vi "GetMethods.vi"(0 "ClassReader in":refnum<class "ClassReader.lvclass">, 5 "error in (no error)":errorcluster) -> (14 "ClassReader out":refnum<class "ClassReader.lvclass">, 15 "Methods":T1[](array[typedef]), 16 "Constructor/CreateIndex":i32, 19 "error out":errorcluster)   [LabVIEW 2014, in "ClassReader.lvclass"]
uses:
  <resource>/Framework/Providers/Open_GDS/ClassProviders/Provider_BaseClassInterface/ClassReader_class/ClassReader.lvclass
  <resource>/Framework/Providers/Open_GDS/ClassProviders/Provider_BaseClassInterface/Types/ClassTypes_MethodType.ctl
  <resource>/Framework/Providers/Open_GDS/ClassProviders/Provider_BaseClassInterface/ClassReader_class/ClassReader.lvclass/ClassReader.ctl
  <resource>/Framework/Providers/Open_GDS/UML/UMLEditor/UMLEditor_VisibilityType.ctl
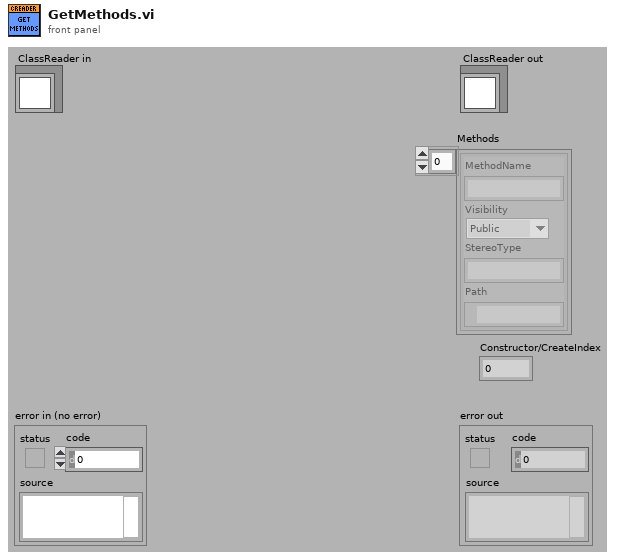
[diagram p1: front panel]
types:
  T1 = typedef "ClassTypes_MethodType.ctl" = cluster{"MethodName":string, "Visibility":enum16{"Public", "Private", "Protected"}, "StereoType":string, "Path":path}
  T2 = typedef "UMLEditor_VisibilityType.ctl" = enum16{"Public", "Private", "Protected"}
  T3 = typedef "Librarian File Info Out.ctl" = cluster{"creation date":u32, "last mod date":u32, "type":string, "creator":string, "LV version":i32, "size":i32, "top level":bool}
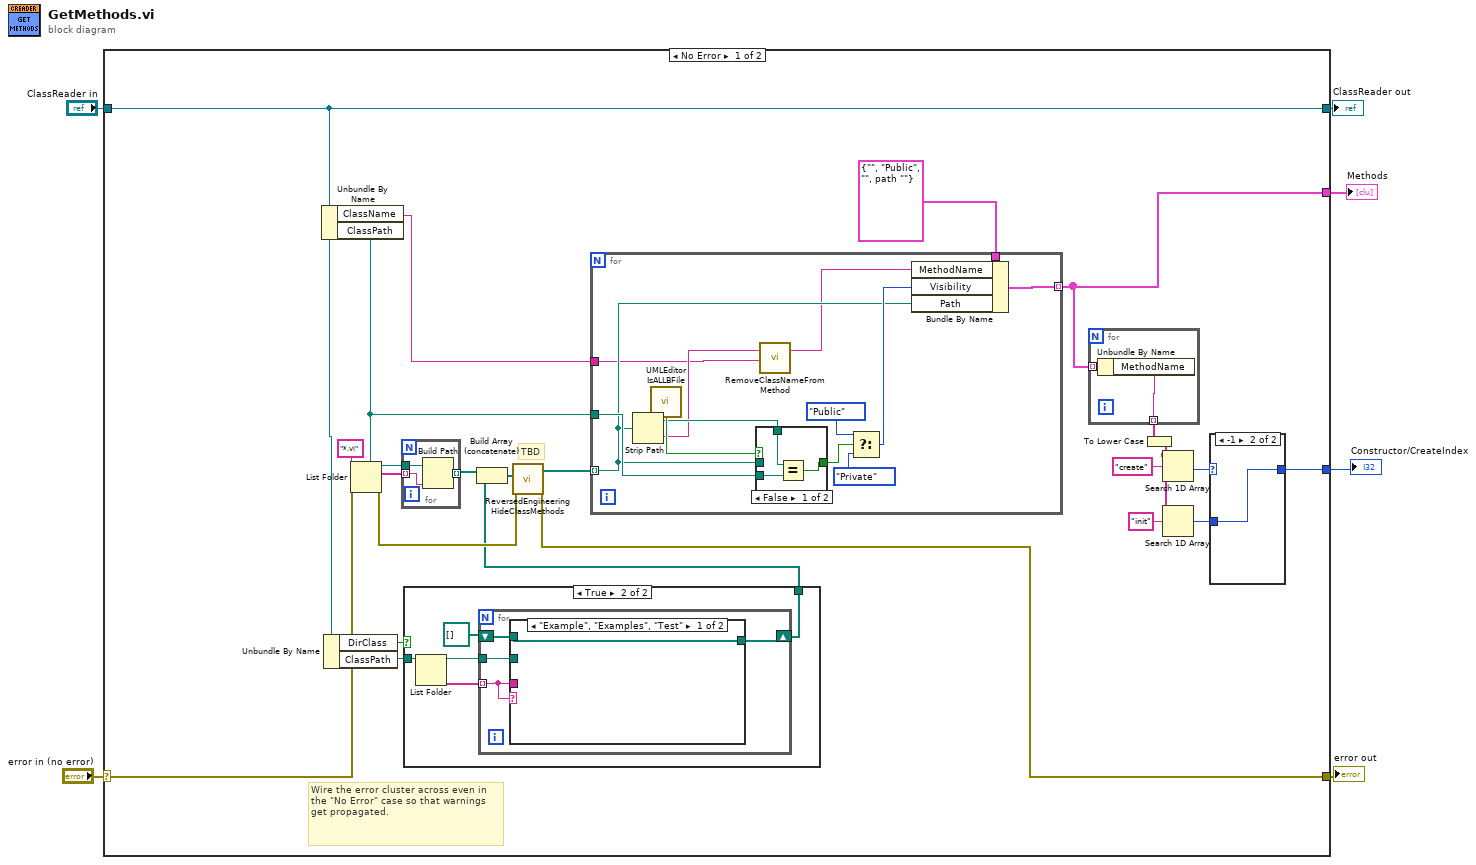
[diagram p0: block diagram]
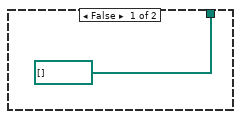
[diagram p3: hidden frame]
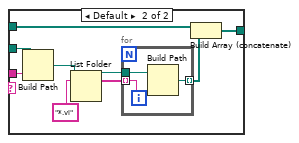
[diagram p4: hidden frame]
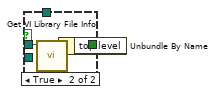
[diagram p5: hidden frame]
diagram:
  n1 = case shown="No Error" "error in (no error)" {
    selector: "error in (no error)" -> [w18 w81]
    tunnel: [w15 w81] -> w5
    tunnel: [w17 w80] -> w3
    tunnel: "ClassReader in" -> [w17 w80]
    tunnel: [w8 _] -> w2
    tunnel: [w7 _] -> w1
    frame No Error {
      # "TBD"
      # "Wire the error cluster across even in the \"No Error\" case so that warnings get propagated."
      n2 = Unbundle By Name(w17) -> ("ClassName"=w22:string, "ClassPath"=w19:path)
      n3 = Unbundle By Name(w17) -> ("DirClass"=w24:bool, "ClassPath"=w23:path)
      n4 = List Folder(path=w19, pattern="*.vi", error in=w18) -> (path out=w30:path, filenames=w29:string[], error out=w26:errorcluster)  [unwired: 1 in, 1 out]
      n5 = for {
        tunnel: w30 -> [w79]
        tunnel: w29 -> [w77] mode=indexing
        tunnel: [w78] -> w28 mode=indexing
        n6 = Build Path(base path=w79, name or relative path=w77) -> (appended path=w78:path)
      }
      n7 = case shown="True" w24 {
        tunnel: w23 -> [_ w40]
        tunnel: [path[] [] w37] -> w21
        frame False {
        }
        frame True {
          n8 = List Folder(path=w40) -> (path out=w39:path, folder names=w38:string[])  [unwired: 3 in, 2 out]
          n9 = for {
            tunnel: w39 -> [w44]
            tunnel: w38 -> [w41] mode=indexing
            shift-right: [w42] -> w37
            shift-left: path[] [] -> [w43]
            n10 = case shown="\"Example\", \"Examples\", \"Test\"" w41 {
              tunnel: w44 -> [_ w51]
              tunnel: w41 -> [_ w50]
              tunnel: w43 -> [w45 w48]
              tunnel: [w45 w47] -> w42
              frame "Example", "Examples", "Test" {
              }
              frame Default {
                n11 = Build Path(base path=w51, name or relative path=w50) -> (appended path=w49:path)
                n12 = List Folder(path=w49, pattern="*.vi") -> (path out=w53:path, filenames=w54:string[])  [unwired: 2 in, 2 out]
                n13 = for {
                  tunnel: w53 -> [w57]
                  tunnel: w54 -> [w55] mode=indexing
                  tunnel: [w56] -> w46 mode=indexing
                  n14 = Build Path(base path=w57, name or relative path=w55) -> (appended path=w56:path)
                }
                n15 = Build Array (concatenate)(w48, w46) -> (w47:path[])
              }
            }
          }
        }
      }
      n16 = Build Array (concatenate)(w28, w21) -> (w20:path[])
      n17 = call <resource>:"ReversedEngineering HideClassMethods.vi"("Item Paths"=w20, "error in (no error)"=w26) -> ("Item Paths filtered"=w27:path[], "error out"=w15:errorcluster)  [unwired: 16 in]
      n18 = for {
        tunnel: w27 -> [w62] mode=indexing
        tunnel: w22 -> [w58]
        tunnel: w19 -> [w68]
        tunnel: T1 {"MethodName"="", "Visibility"=enum."Public", "StereoType"="", "Path"=path ""} ("Method") -> [w64]
        tunnel: [w61] -> w8 mode=indexing
        n19 = Strip Path(path=w62) -> (stripped path=w69:path, name=w60:string)
        n20 = call <resource>:"UMLEditor IsALLBFile.vi"("path"=w69) -> ("path to VI library?"=w70:bool)
        n21 = case shown="False" w70 {
          tunnel: [w71 w75] -> w67
          tunnel: w62 -> [_ w74]
          tunnel: w69 -> [w73 _]
          tunnel: w68 -> [w72 _]
          frame False {
            n22 = Equal?(x=w73, y=w72) -> (x = y?=w71:bool)
          }
          frame True {
            n23 = call <vilib>:"Get VI Library File Info.vi"("path"=w74) -> ("file information"=w76:T3)  [unwired: 9 in, 1 out]
            n24 = Unbundle By Name(w76) -> ("top level"=w75:bool)
          }
        }
        n25 = call <resource>:"RemoveClassNameFromMethod.vi"("MethodVINameIn"=w60, "ClassName"=w58) -> ("MethodVINameOut"=w59:string)  [unwired: 17 in]
        n26 = Select(t=UMLEditor_VisibilityType."Public" ("Enum"), s=w67, f=UMLEditor_VisibilityType."Private" ("Enum")) -> (s? t:f=w63:T2)
        n27 = Bundle By Name(cluster=w64, "MethodName"=w59, "Visibility"=w63, "Path"=w62) -> (w61:T1)
      }
      n28 = for {
        tunnel: w8 -> [w34] mode=indexing
        tunnel: [w33] -> w14 mode=indexing
        n29 = Unbundle By Name(w34) -> ("MethodName"=w33:string)
      }
      n30 = To Lower Case(string=w14) -> (all lower case string=w12:string[])
      n31 = Search 1D Array(1D array=w12, element="create") -> (index of element=w10:i32)  [unwired: 1 in]
      n32 = Search 1D Array(1D array=w12, element="init") -> (index of element=w9:i32)  [unwired: 1 in]
      n33 = case shown="-1" w10 {
        selector: w10 -> [w31 _]
        tunnel: [w31 w32] -> w7
        tunnel: w9 -> [_ w32]
        frame Default {
        }
        frame -1 {
        }
      }
    }
    frame Error {
    }
  }
  "error out" <- w5
  "ClassReader out" <- w3
  "Methods" <- w2
  "Constructor/CreateIndex" <- w1
